vi "DSF.Memory.Buffer.Get Channel Count.vi"(8 "error in (no error)":errorcluster, 11 "Buffer in":refnum<class "DSF.Memory.Buffer.lvclass">) -> (0 "error out":errorcluster, 2 "channel count":u64 format="%d channels", 3 "Buffer out":refnum<class "DSF.Memory.Buffer.lvclass">)   [LabVIEW 2016, in "DSF.Memory.lvlib" / "DSF.Memory.Buffer.lvclass"]
uses:
  DSF.Memory.Buffer.lvclass
  DSF.Memory.Buffer.lvclass/DSF.Memory.Buffer.ctl
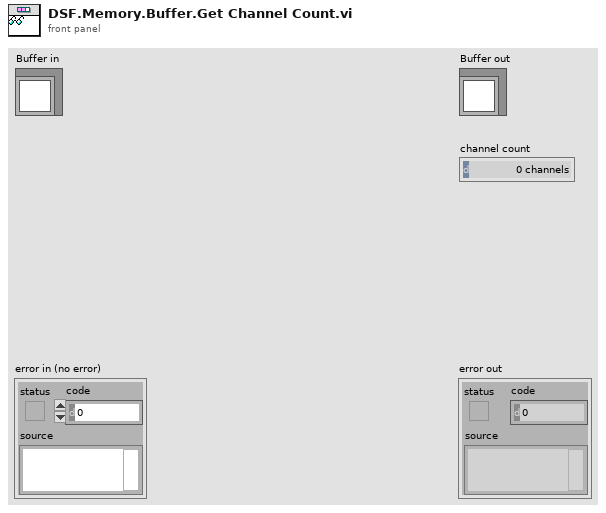
[diagram p1: front panel]
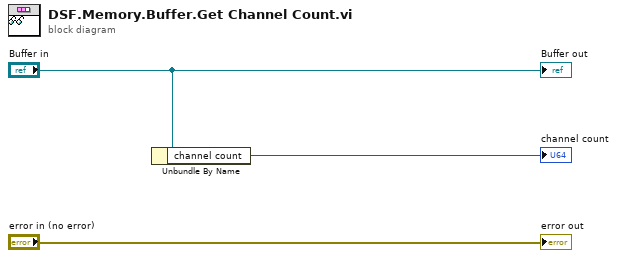
[diagram p0: block diagram]
diagram:
  n1 = Unbundle By Name("Buffer in") -> ("channel count"=→"channel count":u64)
  "error out" <- "error in (no error)"
  "Buffer out" <- "Buffer in"
